vi "Write.vi"(5 "TDMS Group in":refnum<class "Group.lvclass">, 8 "error in (no error)":errorcluster, 9 "Group Properties":refnum<class "Variant.lvclass">, 10 "Channels":refnum<class "Channel.lvclass">[](array[class]), 11 "Group Name":string) -> (0 "error out":errorcluster, 3 "TDMS Group out":refnum<class "Group.lvclass">)   [LabVIEW 2020, in "TDMS.lvlib" / "Group.lvclass"]
doc: "Write Group Name, Channels and Properties."
uses:
  Group.lvclass
  TDMS Channel/Channel.lvclass
  PPL/HDH.Data.Generic.lvlibp/Generic Data/Variant/Variant.lvclass
  Group.lvclass/Group.ctl
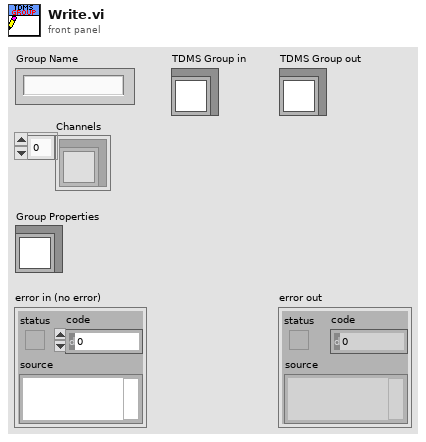
[diagram p1: front panel]
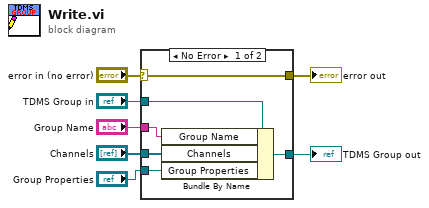
[diagram p0: block diagram]
diagram:
  n1 = case shown="No Error" "error in (no error)" {
    selector: "error in (no error)" -> [w13 w14]
    tunnel: [w13 w14] -> w6
    tunnel: [w11 w15] -> w4
    tunnel: "TDMS Group in" -> [w12 w15]
    tunnel: "Group Name" -> [w10 _]
    tunnel: "Channels" -> [w9 _]
    tunnel: "Group Properties" -> [w8 _]
    frame No Error {
      n2 = Bundle By Name(cluster=w12, "Group Name"=w10, "Channels"=w9, "Group Properties"=w8) -> (w11:refnum<class "Group.lvclass">)
    }
    frame Error {
    }
  }
  "error out" <- w6
  "TDMS Group out" <- w4
